vi "draw.vi"(8 "error in (no error)":errorcluster, 11 "afRectangle in":refnum<class "afRectangle.lvclass">) -> (0 "error out":errorcluster, 3 "afRectangle out":refnum<class "afRectangle.lvclass">)   [LabVIEW 2017, in "afRectangle.lvclass"]
uses:
  afRectangle.lvclass
  ConsoleOut/Print Options.ctl
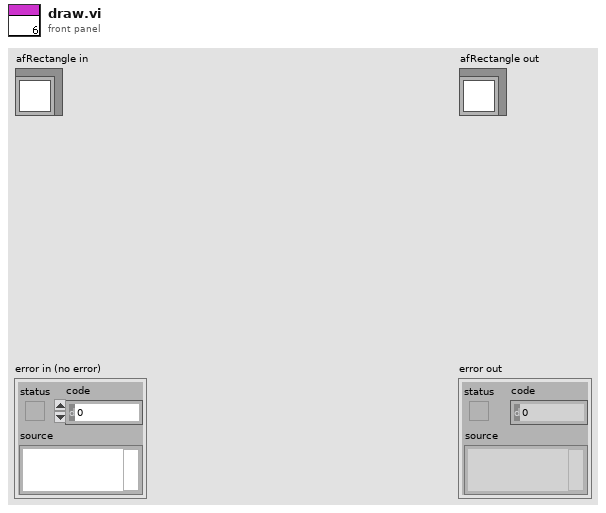
[diagram p1: front panel]
types:
  T1 = typedef "Print Options.ctl" = enum16{"Create", "Get Reference", "Print", "Print Header", "Close"}
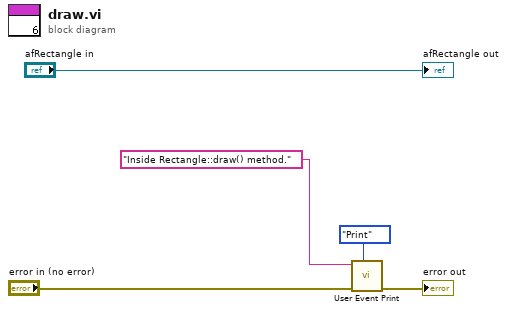
[diagram p0: block diagram]
diagram:
  n1 = call "User Event Print.vi"("Options"=Print_Options."Print", "error in (no error)"="error in (no error)", "String to Print"="Inside Rectangle::draw() method." ("message")) -> ("error out"=→"error out":errorcluster)  [unwired: 7 in, 1 out]
  "afRectangle out" <- "afRectangle in"
